vi "PathDrawerMain.vi"() -> ()   [LabVIEW 2017]
uses:
  Shared/PathFileData.ctl
  Shared/RobotNeededPathData.ctl
panel:
  in  "Tab Control":enum32{"Path", "Load/Save"}(tab)
  in  "SlowSpeed":dbl=15.0 format="%#_13g"
  in  "SlowDistanceAtEnd":dbl=12.0 format="%#_13g"
  in  "Speed/Curve":dbl=1.8 format="%#_13g"
  in  "DriveBackwards?":bool
  in  "Lookahead":dbl=15.0
  out "Points (in)":cluster{dbl, dbl}[](array[cluster])=[{10.226685796269727, 128.2984218077475}, {15.522939790252737, 129.12001667538078}, {20.706046011417115, 130.03734410344734}, {25.64419820355277, 131.16153224586634}, {30.166489666811938, 132.63728713251658}, {34.03433393234178, 134.66614678695453}, {37.84312996845399, 137.57541844379503}, {41.613199324830866, 141.06936663595954}, {45.358528302145274, 144.94685599230576}, {49.089111176273455, 149.06887095200779}, {52.81248148388562, 153.3359781588411}, {56.53509433279494, 157.67228944092315}, {60.26328881425947, 162.01308055786865}, {64.00426865578318, 166.29432163323958}, {67.7673029921362, 170.44235444566638}, {71.56524618905358, 174.36196698028664}, {75.41661103612846, 177.92096482194324}, {79.3485578107416, 180.92876767612321}, {83.40129053463254, 183.10555843063264}, {88.0121428846403, 184.52243744962843}, {92.95651186406619, 185.43308931394066}, {98.06376666039486, 186.00922465888777}, {103.18969721381382, 186.36840832003176}, {108.19306201885799, 186.59306844321625}, {112.91282926380357, 186.74384781305636}, {117.14203730272597, 186.86944045911048}]
  in  "Points":cluster{dbl, dbl}[](array[cluster])=[{35.0, 207.0}, {61.0, 206.0}, {110.0, 143.0}, {150.0, 144.0}]
  in  "Roundedness":dbl(slide)=0.8606565656565657 scale=0.6..0.997
  in  "Length":dbl=29.0
  in  "Width":dbl=32.0
  in  "CenterRotOffset":dbl=10.5
  in  "PointSpacing":dbl=6.0 min=1.0 format="%#_13g"
  in  "StartingPosition":enum16{"1", "2", "3", "4", "No Preset"}(ring)=enum."3"
  in  "Flip Path":bool
  in  "MaxVel":dbl=130.0 format="%#_13g"
  in  "MaxAccel":dbl=50.0 format="%#_13g"
  in  "ExportAllToRobot":bool
  in  "LocalTempPaths":i32(listbox)
  out "standard output":string
  in  "SaveToLocal":bool
  in  "LoadFromLocal":bool
  in  "ExportToRobot":bool
  in  "LoadAllFromRobot":bool
  in  "LocalPaths":i32(listbox)=3
  out "standard error":string="NI Linux Real-Time (run mode)\n\nLog in with your NI-Auth credentials.\n\n"
  in  "LocalFileNames":string[](array[string])=["1A.txt", "1B.txt", "1C.txt", "3A.txt", "4B.txt"]
  in  "Stop":bool
  out "Path Drawer":T1(plugin-control)
  # "Includes bumpers"
  # "Relative to outside face of\nback bumber of robot"
  # "INSTRUCTIONS"
  # "The red line is the path that the robot recieves. Everything else is to help create that path\n\nUse the multi-line tool to draw a path. Double click to stop drawing.\nHover over a node and press backspace to remove it.\nPress I to insert a new node (at the end of the path only, for now)\n\nUse the contols to input robot width, height, and center of rotation offset,\nHow far apart the points in the \"real world units\" path are,\nWhether the robot travels on the left or right of your green lines, and\nthe roundedness of the path. (Note: point spacing affects roundedness)\n\nYou can manually edit the green node's location in the path with the Points array,\nor drag the nodes on the image\n\nPress Export To File and enter the file name (no extension) to save the path to a file in the\nThisVIsDirectory\\Paths\\ folder\n\nIf you acidentally clear your path press Z quickly to get it back"
  # "Responses of CMDs run"
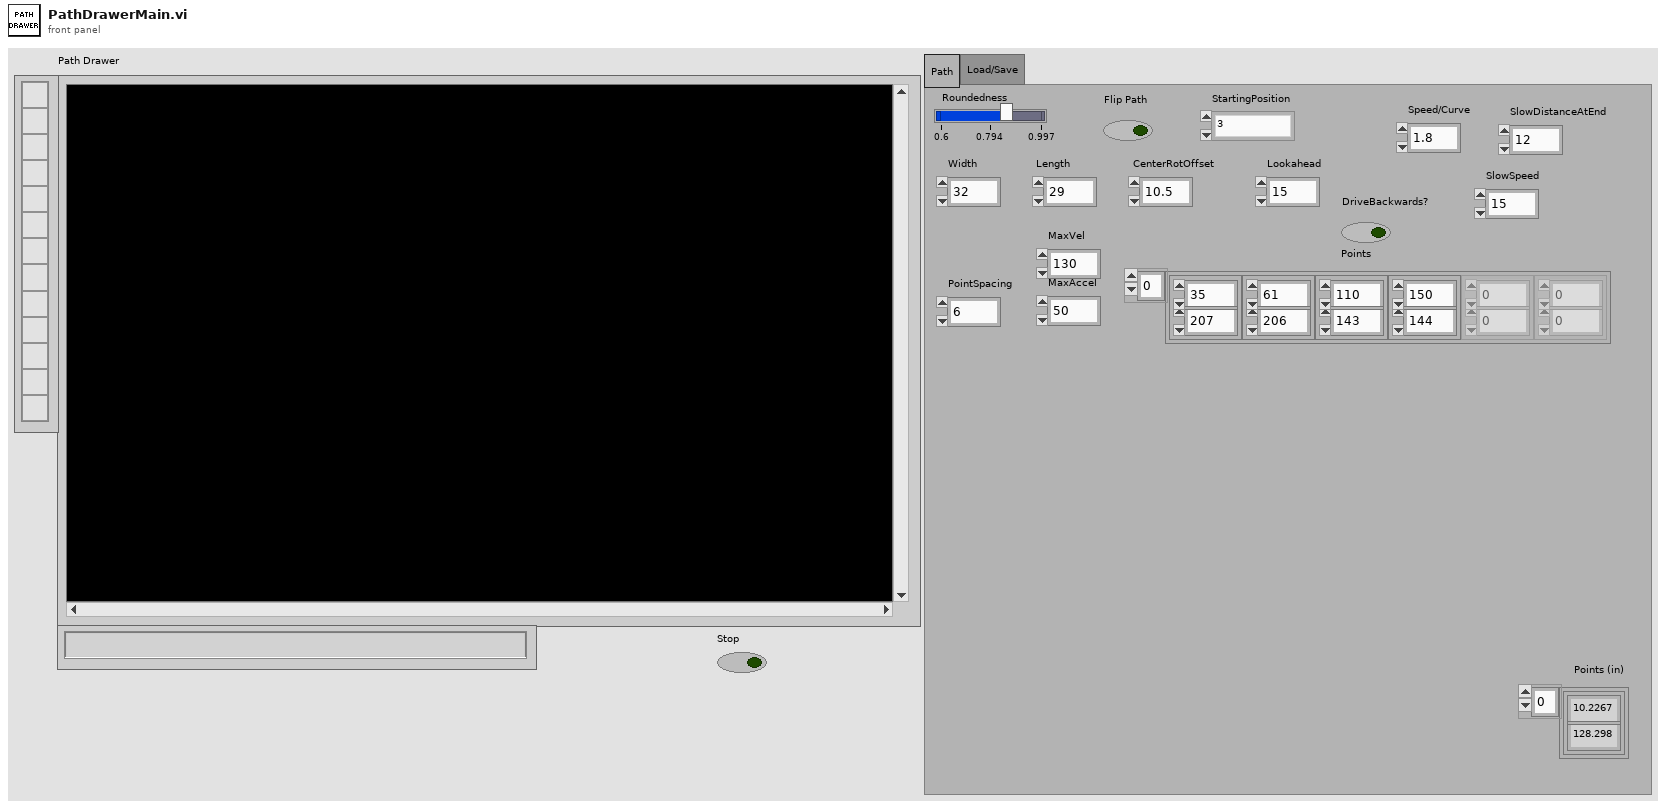
[diagram p1: front panel]
types:
  T1 = typedef "IMAQ Image.ctl" = refnum<image>
  T2 = typedef "Image Type" = u32
  T3 = enum16{"open", "replace", "create", "open or create", "replace or create", "replace or create with confirmation"}
  T4 = cluster{"Global Rectangle":i32[], "Contours":cluster{"Contour Type":u32, "ROI Type":u32, "Points":i32[]}[]}
  T5 = cluster{"Contour Type":u32, "ROI Type":u32, "Points":i32[]}[]
  T6 = cluster{"Contour Type":u32, "ROI Type":u32, "Points":i32[]}
  T7 = typedef "PathFileData.ctl" = cluster{"RobotNeeded":T8, "Meta":cluster{"Path (px)":cluster{i32, i32}[], "RobotWidth":dbl, "RobotLength":dbl, "CenterOfRotYOffset":dbl, "Roundedness":dbl, "StartingPositionPreset":u32, "PathName":string}}
  T8 = typedef "RobotNeededPathData.ctl" = cluster{"Path":cluster{dbl, dbl}[], "MaxVel":dbl, "MaxAccel":dbl, "Backwards?":bool, "PointSpacing":dbl, "LookaheadDist":dbl, "Speed/Curve":dbl, "SlowDistanceAtEnd":dbl, "SlowSpeed":dbl}
  T9 = cluster{"Path (px)":cluster{i32, i32}[], "RobotWidth":dbl, "RobotLength":dbl, "CenterOfRotYOffset":dbl, "Roundedness":dbl, "StartingPositionPreset":u32, "PathName":string}
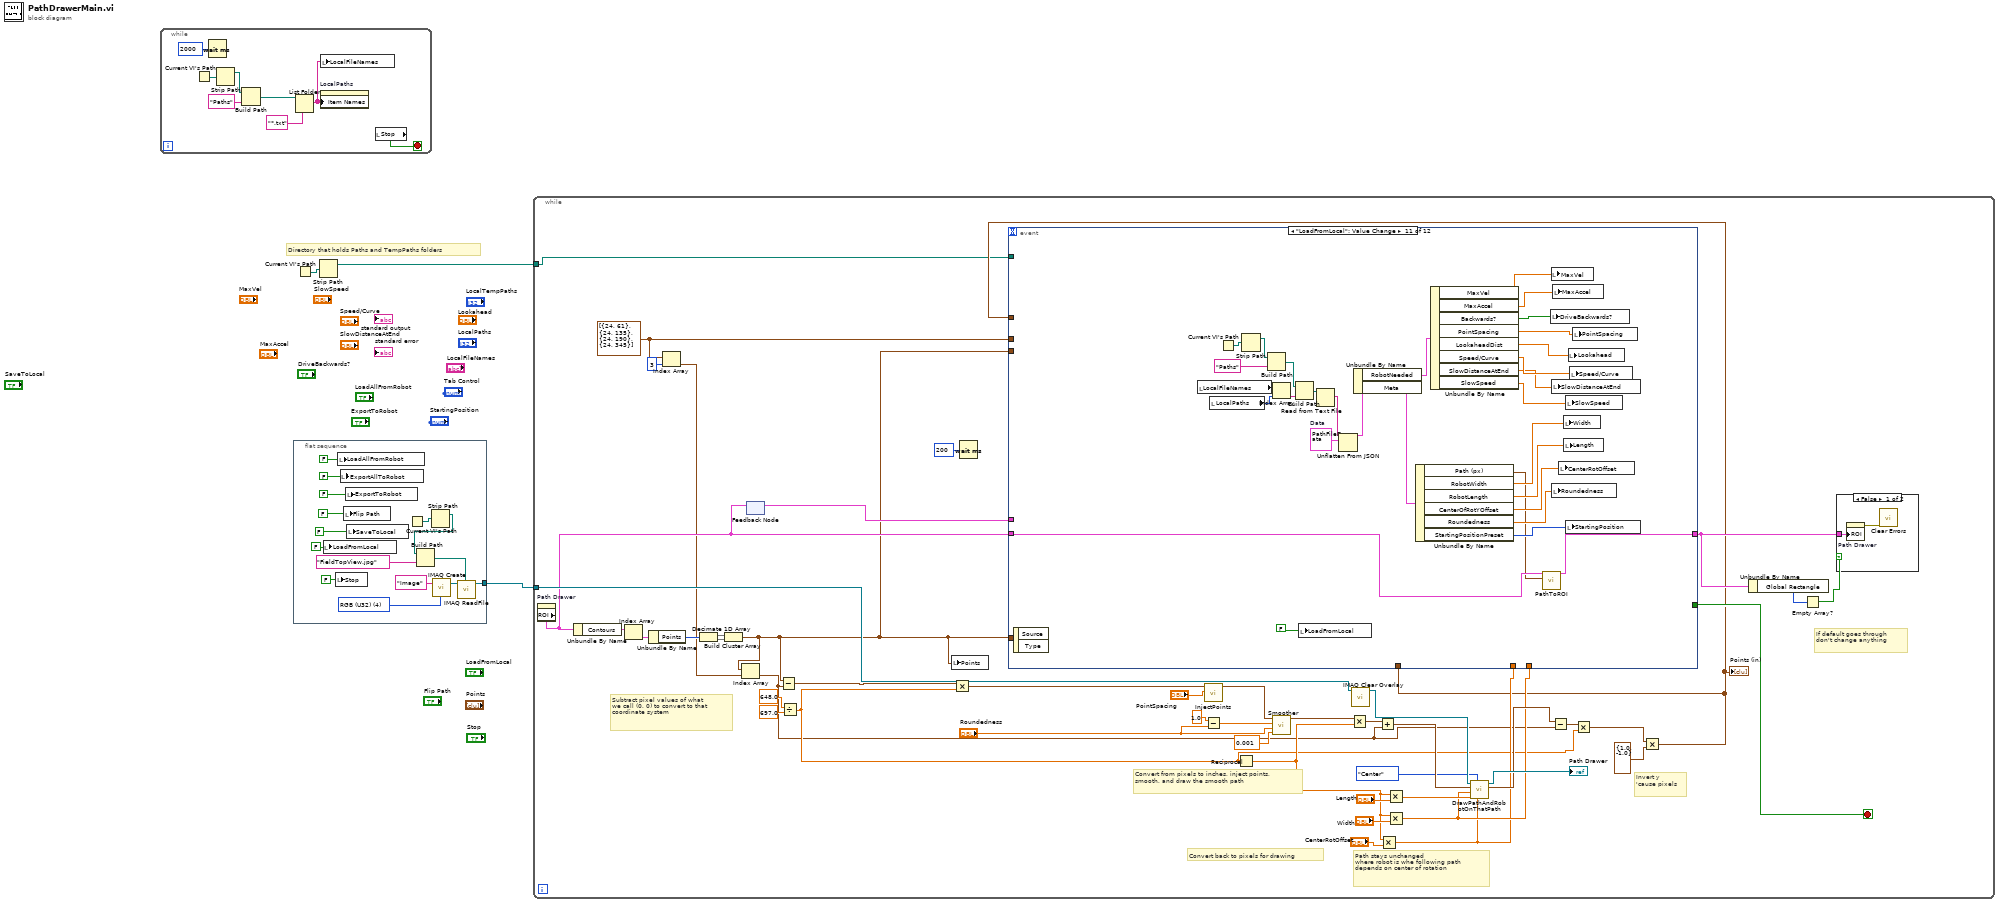
[diagram p0: block diagram]
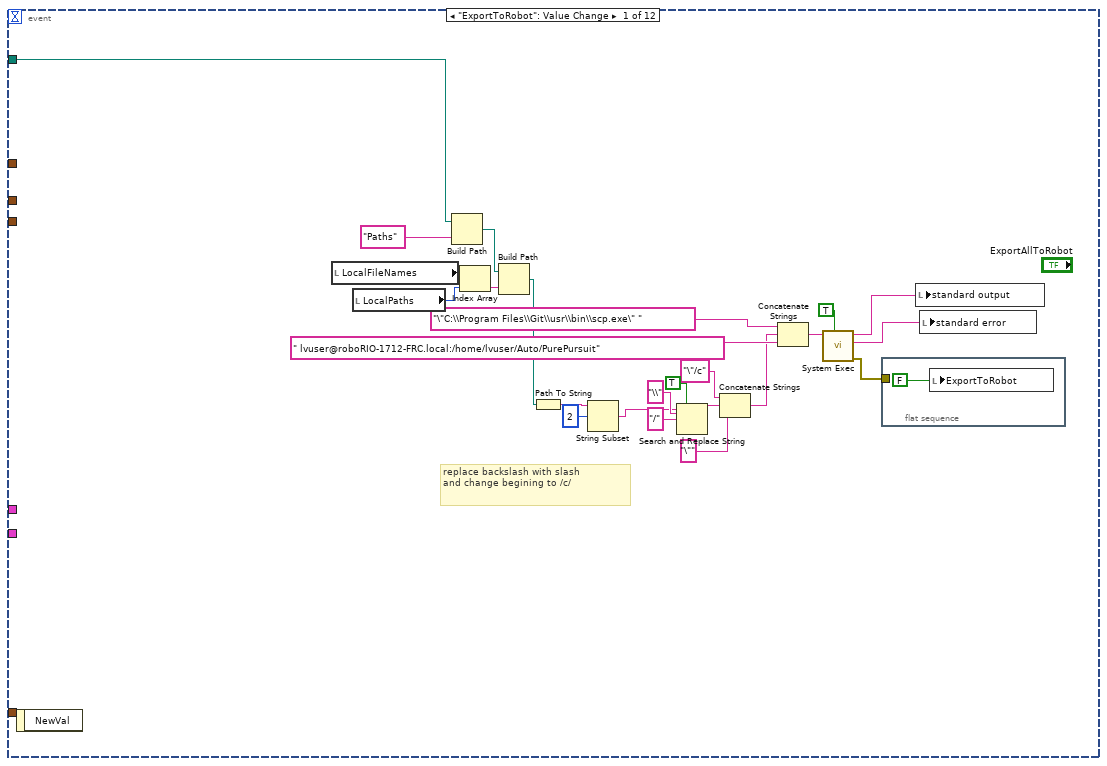
[diagram p3: hidden frame]
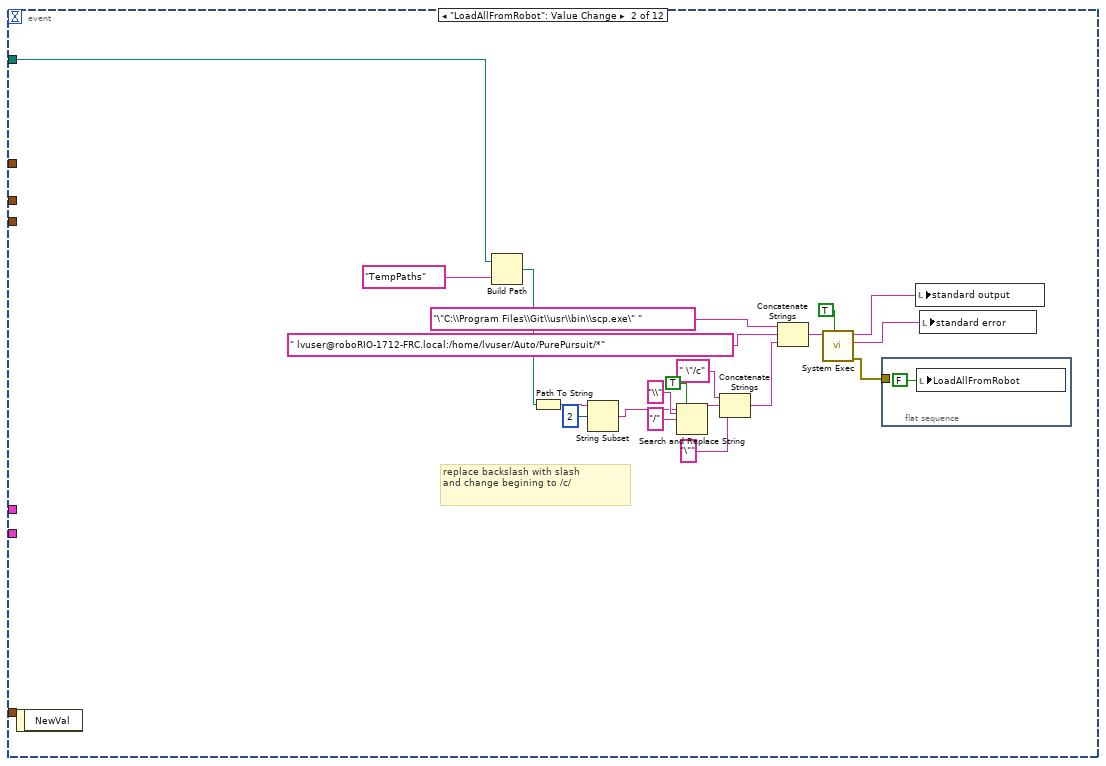
[diagram p4: hidden frame]
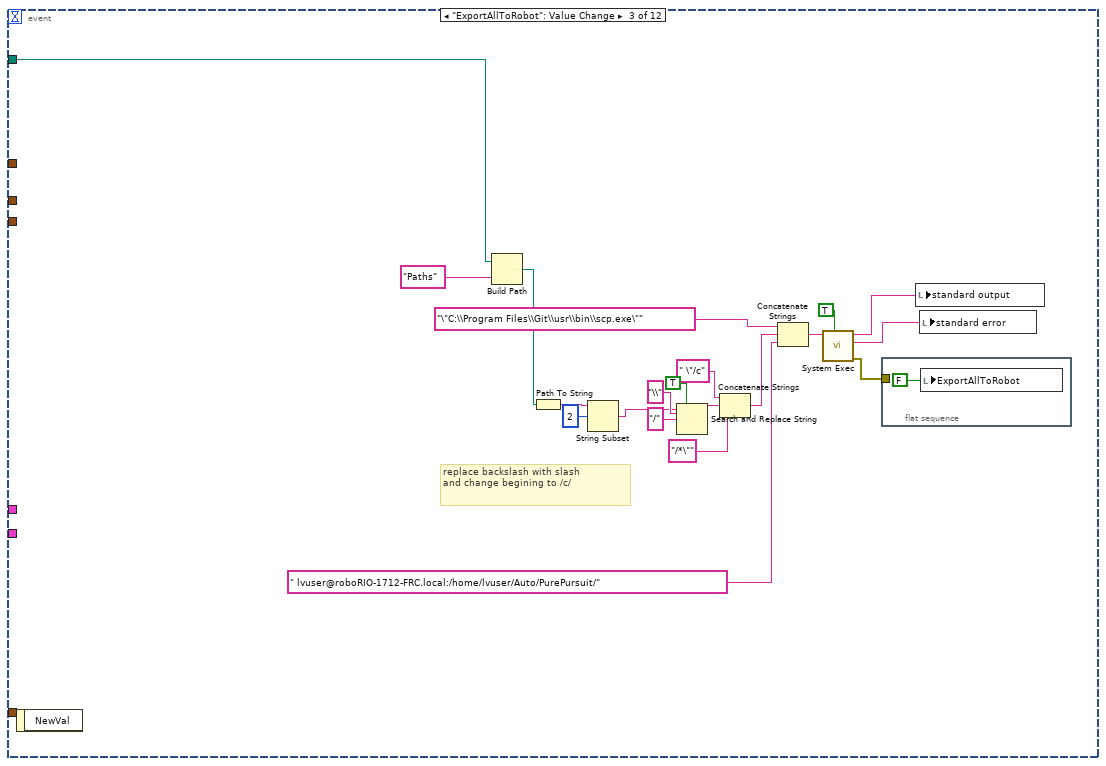
[diagram p5: hidden frame]
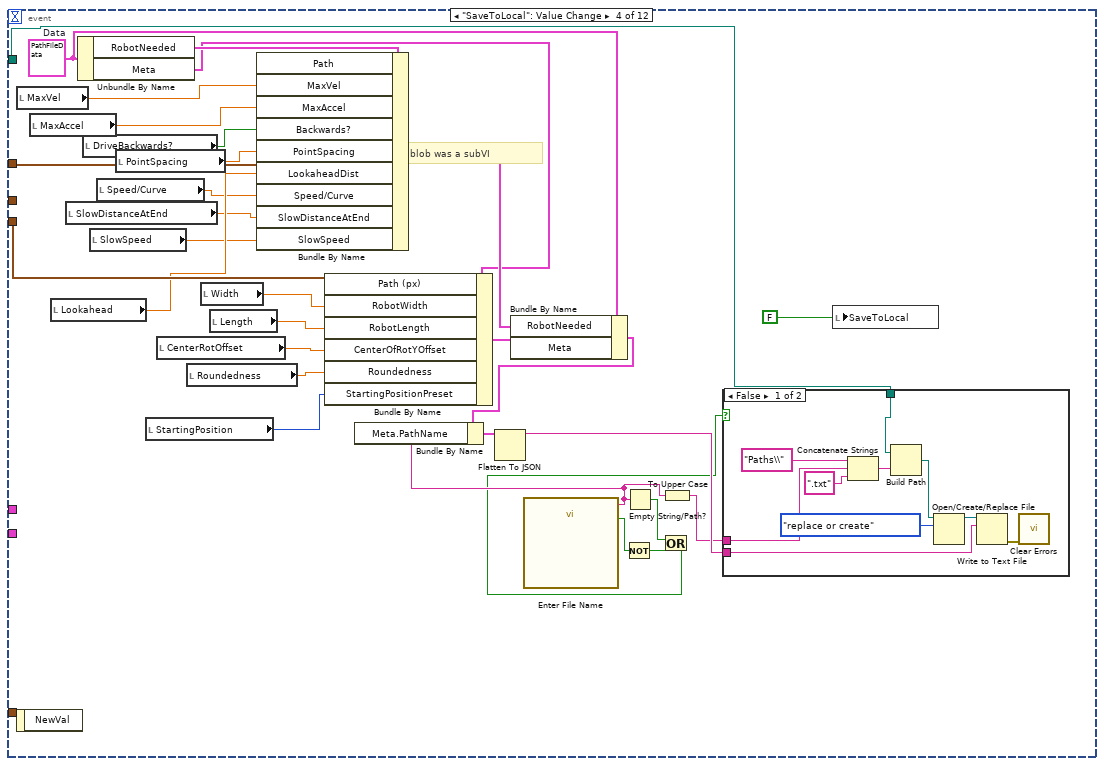
[diagram p6: hidden frame]
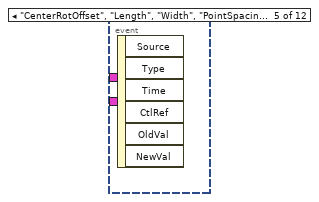
[diagram p8: hidden frame]
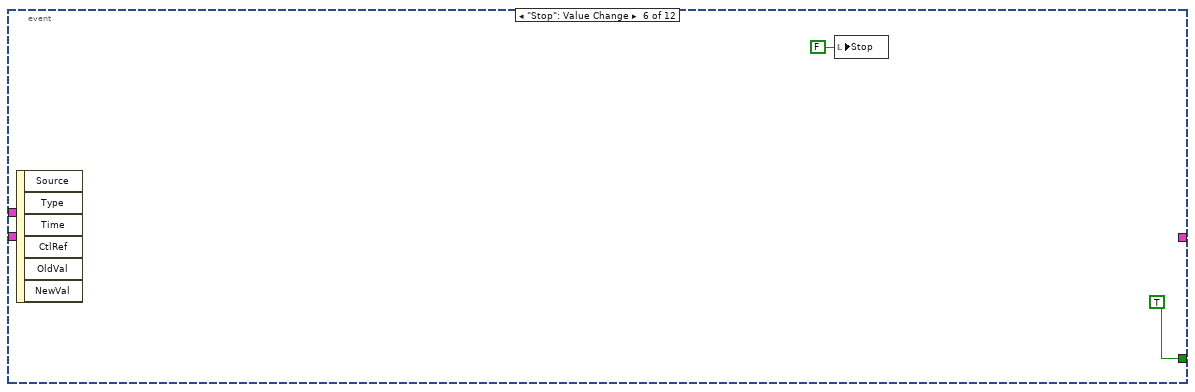
[diagram p9: hidden frame]
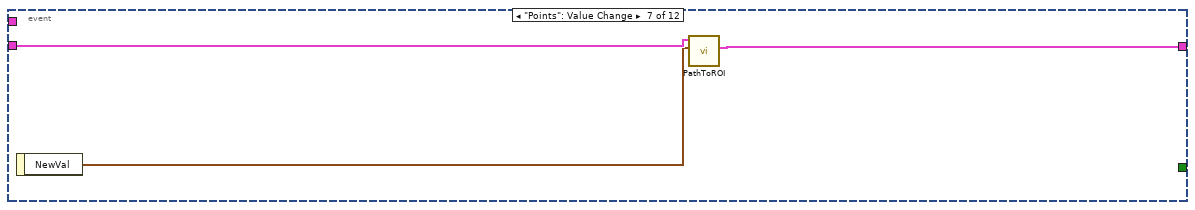
[diagram p10: hidden frame]
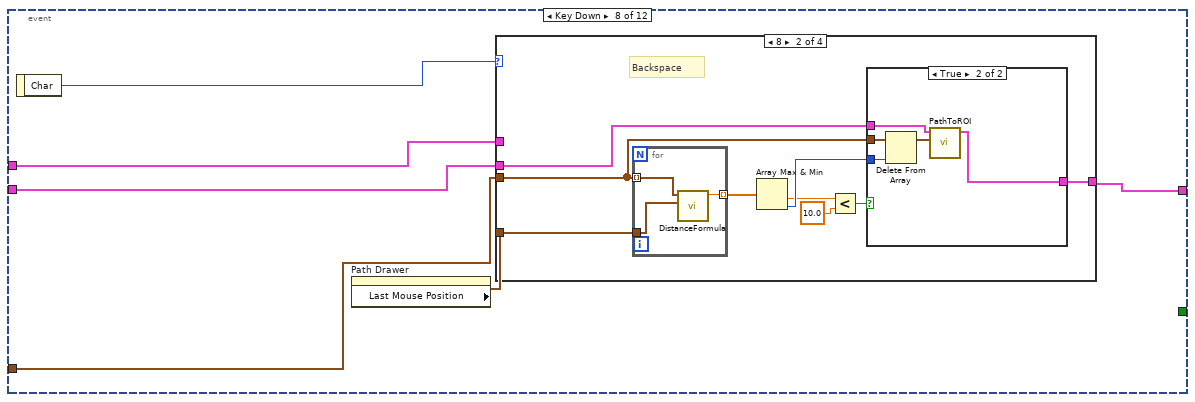
[diagram p11: hidden frame]
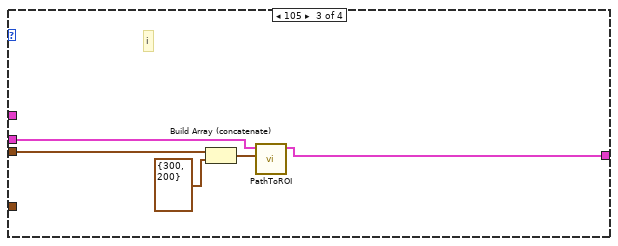
[diagram p14: hidden frame]
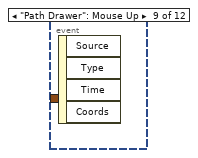
[diagram p16: hidden frame]
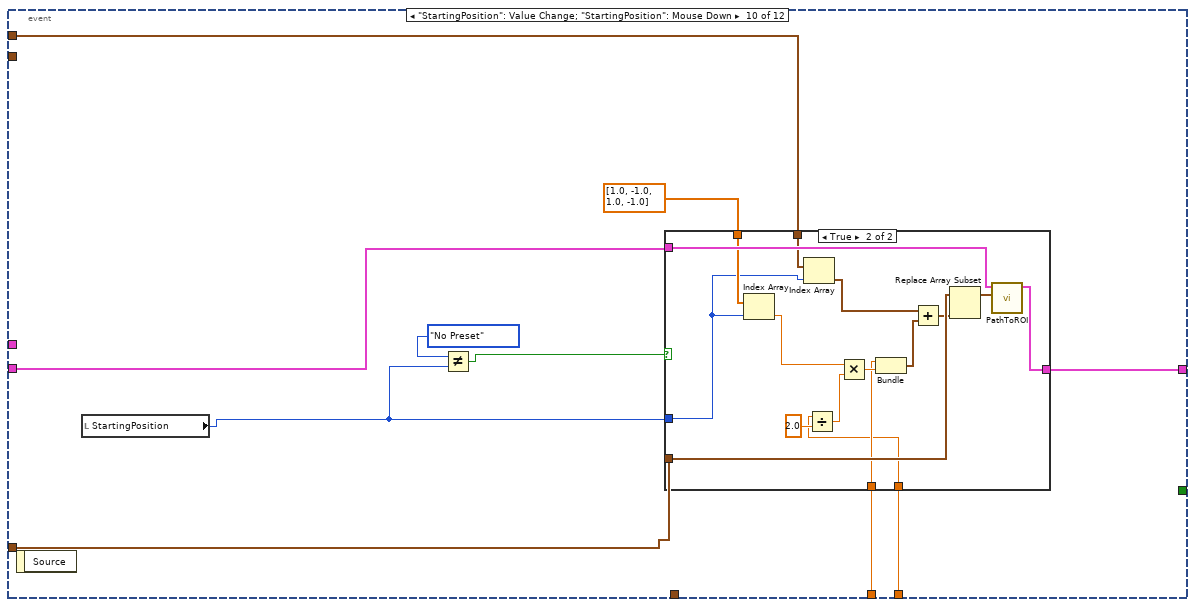
[diagram p17: hidden frame]
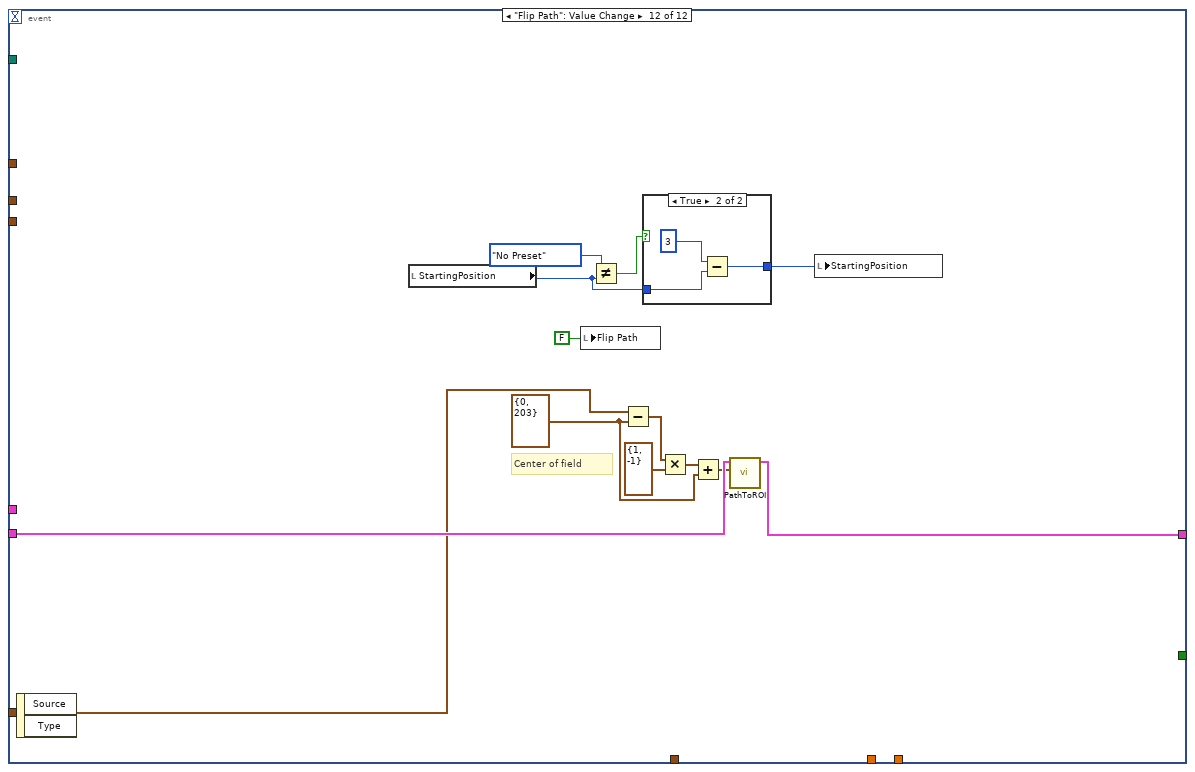
[diagram p19: hidden frame]
diagram:
  # "Directory that holds Paths and TempPaths folders"
  n1 = while {
    stop <- w10 stop-if-true
    n2 = Current VI's Path() -> (path=w5:path)
    n3 = Wait (ms)(milliseconds to wait=u32 2000) -> ()  [unwired: 1 out]
    n4 = Strip Path(path=w5) -> (stripped path=w4:path)  [unwired: 1 out]
    n5 = Build Path(base path=w4, name or relative path="Paths") -> (appended path=w7:path)
    n6 = List Folder(path=w7, pattern="*.txt") -> (filenames=w9:string[])  [unwired: 2 in, 3 out]
    n7 = local write "LocalFileNames"(w9) -> ()
    n8 = property on="LocalPaths" class="LstBox (strict)"("Item Names"=w9) -> ()  [unwired: 2 in, 2 out]
    n9 = local read "Stop"() -> (w10:bool)
  }
  n10 = flat-sequence {
    tunnel: [w21] -> w3
    frame #0 {
      w23 = T2 4 items=["Grayscale (U8)", "Grayscale (I16)", "Grayscale (SGL)", "Complex (CSG)", "RGB (U32)", "HSL (U32)", "RGB (U64)", "Grayscale (U16)"] ("Image Type")
      n11 = local write "LoadFromLocal"(FALSE ("Export To File")) -> ()
      n12 = local write "Stop"(FALSE ("Stop")) -> ()
      n13 = local write "LoadAllFromRobot"(FALSE ("Export To File")) -> ()
      n14 = local write "ExportAllToRobot"(FALSE ("Export To File")) -> ()
      n15 = local write "Flip Path"(FALSE ("Export To File")) -> ()
      n16 = local write "ExportToRobot"(FALSE ("Export To File")) -> ()
      n17 = local write "SaveToLocal"(FALSE ("Export To File")) -> ()
      n18 = Current VI's Path() -> (path=w15:path)
      n19 = Strip Path(path=w15) -> (stripped path=w14:path)  [unwired: 1 out]
      n20 = Build Path(base path=w14, name or relative path="FieldTopView.jpg") -> (appended path=w25:path)
      n21 = call "IMAQ Create"("Image Name"="Image", "Image Type"=w23) -> ("New Image"=w22:T1)  [unwired: 3 in, 1 out]
      n22 = call "IMAQ ReadFile"("File Path"=w25, "Image"=w22) -> ("Image Out"=w21:T1)  [unwired: 5 in, 4 out]
    }
  }
  n23 = Current VI's Path() -> (path=w2:path)
  n24 = Strip Path(path=w2) -> (stripped path=w1:path)  [unwired: 1 out]
  n25 = while {
    tunnel: w3 -> [w67]
    tunnel: w1 -> [w30]
    stop <- w40 stop-if-true
    w29 = cluster{u32, u32}[] [{24, 61}, {24, 135}, {24, 190}, {24, 345}]
    # "Invert y\n'cause pixels"
    # "Path stays unchanged\nwhere robot is whe following path\ndepends on center of rotation"
    # "Convert back to pixels for drawing"
    # "If default goes through\ndon't change anything"
    # "Convert from pixels to inches, inject points,\nsmooth, and draw the smooth path"
    # "Subtract pixel values of what\nwe call (0, 0) to convert to that\ncoordinate system"
    n26 = property on="Path Drawer" class="ImageControl"() -> ("ROI"=w34:T4)  [unwired: 2 in, 2 out]
    n27 = Unbundle By Name(w34) -> ("Contours"=w73:T5)
    n28 = Index Array(array=w73) -> (element=w68:T6)  [unwired: 1 in]
    n29 = Unbundle By Name(w68) -> ("Points"=w62:i32[])
    n30 = Index Array(array=w29, index=3) -> (element=w27:cluster{u32, u32})
    n31 = Decimate 1D Array(w62) -> (w72:i32[], w71:i32[])
    n32 = Build Cluster Array(w72, w71) -> (w32:cluster{i32, i32}[])
    n33 = Index Array(array=w32) -> ()  [unwired: 1 in, 1 out]
    n34 = feedback-in #1(w34) -> ()
    n35 = feedback #1() -> (w49:T4)  [unwired: 1 in]
    n36 = Subtract(x=w32, y=w27) -> (x-y=w63:cluster{u32, u32}[])
    n37 = Divide(x=648.0, y=697.0) -> (x/y=w35:dbl)
    n38 = local write "Points"(w32) -> ()
    n39 = Multiply(x=w63, y=w35) -> (x*y=w50:cluster{dbl, dbl}[])
    n40 = Wait (ms)(milliseconds to wait=u32 200) -> ()  [unwired: 1 out]
    n41 = call "InjectPoints.vi"("Distance"="PointSpacing", "Path"=w50) -> ("Path out"=w65:cluster{dbl, dbl}[])  [unwired: 9 in]
    n42 = Subtract(x=1.0, y="Roundedness") -> (x-y=w60:dbl)
    n43 = Reciprocal(x=w35) -> (1/x=w47:dbl)
    n44 = call "Smoother.vi"("tolerance"=0.001, "B"="Roundedness", "A"=w60, "Path"=w65) -> ("SmoothPath"=w55:cluster{dbl, dbl}[])  [unwired: 7 in]
    n45 = Multiply(x=w55, y=w47) -> (x*y=w64:cluster{dbl, dbl}[])
    n46 = call "IMAQ Clear Overlay"("Image"=w67) -> ("Image Out"=w44:T1)  [unwired: 9 in, 1 out]
    n47 = Add(x=w64, y=w27) -> (x+y=w43:cluster{dbl, dbl}[])
    n48 = Multiply(x=w47, y="CenterRotOffset") -> (x*y=w38:dbl)
    n49 = Multiply(x=w47, y="Length") -> (x*y=w42:dbl)
    n50 = Multiply(x=w47, y="Width") -> (x*y=w39:dbl)
    n51 = call "DrawPathAndRobotOnThatPath.vi"("CenterOfRotYOffset (px)"=w38, "PathMode"=enum16{"Left", "Right", "Center"}."Center", "RobotLength (px)"=w42, "RobotWidth (px)"=w39, "Path (px)"=w43, "Image In"=w44) -> ("NewPath (px)"=w45:cluster{dbl, dbl}[], "Image Out"=→"Path Drawer":T1)  [unwired: 4 in]
    n52 = Subtract(x=w45, y=w27) -> (x-y=w51:cluster{dbl, dbl}[])
    n53 = Multiply(x=w51, y=w35) -> (x*y=w37:cluster{dbl, dbl}[])
    n54 = Multiply(x=w37, y=cluster{dbl, dbl} {1.0, -1.0}) -> (x*y=w31:cluster{dbl, dbl}[])
    "Points (in)" <- w31
    n55 = event shown="[10] \"LoadFromLocal\": Value Change" {
      selector: _ -> [_ _ _ _ _ _ _ _ _ _ _ _]
      dyn-events: _ -> [_ _ _ _ _ _ _ _ _ _ _ _]
      timeout: _ -> [_ _ _ _ _ _ _ _ _ _ _ _]
      tunnel: w34 -> [_ _ _ _ _ _ w188 w194 _ w228 w260 w287]
      tunnel: [_ _ _ _ _ _ w187 w191 _ w229 w274 w286] -> w33
      tunnel: w31 -> [_ _ _ _ _ _ _ _ _ _ _ _]
      tunnel: w49 -> [_ _ _ _ _ _ _ w190 _ _ _ _]
      tunnel: w32 -> [_ _ _ _ _ _ _ w189 _ w223 _ w281]
      tunnel: w38 -> [_ _ _ _ _ _ _ _ _ w225 _ _]
      tunnel: w39 -> [_ _ _ _ _ _ _ _ _ w224 _ _]
      tunnel: [_ _ _ _ _ TRUE ("Stop") _ _ _ _ _ _] -> w40
      tunnel: w32 -> [_ _ _ w157 _ _ _ _ _ _ _ _]
      tunnel: w31 -> [_ _ _ w156 _ _ _ _ _ _ _ _]
      tunnel: w30 -> [w76 w101 w122 w149 _ _ _ _ _ _ _ _]
      tunnel: w29 -> [_ _ _ _ _ _ _ _ _ w220 _ _]
      event "ExportToRobot": Value Change {
        # "replace backslash with slash\nand change begining to /c/"
        n56 = event-data() -> ()  [unwired: 1 in, 1 out]
        n57 = local read "LocalFileNames"() -> (w83:string[])
        n58 = local read "LocalPaths"() -> (w84:i32)
        n59 = Build Path(base path=w76, name or relative path="Paths") -> (appended path=w86:path)
        n60 = Index Array(array=w83, index=w84) -> (element=w85:string)
        n61 = Build Path(base path=w86, name or relative path=w85) -> (appended path=w81:path)
        n62 = Path To String(path=w81) -> (string=w92:string)
        n63 = String Subset(string=w92, offset (0)=2) -> (substring=w90:string)  [unwired: 1 in]
        n64 = Search and Replace String(replace all?=TRUE ("replace all? (F)"), input string=w90, search string="\\", replace string="/" ("replace string (\"\")")) -> (result string=w89:string)  [unwired: 4 in, 3 out]
        n65 = Concatenate Strings("\"/c" ("string"), w89, "\"" ("string")) -> (w87:string)
        n66 = Concatenate Strings("\"C:\\Program Files\\Git\\usr\\bin\\scp.exe\" " ("command line"), w87, " lvuser@roboRIO-1712-FRC.local:/home/lvuser/Auto/PurePursuit" ("string")) -> (w96:string)
        n67 = call <vilib>:"System Exec.vi"("wait until completion? (T)"=TRUE, "command line"=w96) -> ("error out"=w79:errorcluster, "standard error"=w77:string, "standard output"=w78:string)  [unwired: 6 in, 1 out]
        n68 = flat-sequence {
          tunnel: w79 -> [_]
          frame #0 {
            n69 = local write "ExportToRobot"(FALSE ("Export To File")) -> ()
          }
        }
        n70 = local write "standard output"(w78) -> ()
        n71 = local write "standard error"(w77) -> ()
      }
      event "LoadAllFromRobot": Value Change {
        # "replace backslash with slash\nand change begining to /c/"
        n72 = event-data() -> ()  [unwired: 1 in, 1 out]
        n73 = Build Path(base path=w101, name or relative path="TempPaths") -> (appended path=w104:path)
        n74 = Path To String(path=w104) -> (string=w114:string)
        n75 = String Subset(string=w114, offset (0)=2) -> (substring=w112:string)  [unwired: 1 in]
        n76 = Search and Replace String(replace all?=TRUE ("replace all? (F)"), input string=w112, search string="\\", replace string="/" ("replace string (\"\")")) -> (result string=w111:string)  [unwired: 4 in, 3 out]
        n77 = Concatenate Strings(" \"/c" ("string"), w111, "\"" ("string")) -> (w102:string)
        n78 = Concatenate Strings("\"C:\\Program Files\\Git\\usr\\bin\\scp.exe\" " ("command line"), " lvuser@roboRIO-1712-FRC.local:/home/lvuser/Auto/PurePursuit/*" ("string"), w102) -> (w118:string)
        n79 = call <vilib>:"System Exec.vi"("wait until completion? (T)"=TRUE, "command line"=w118) -> ("error out"=w107:errorcluster, "standard error"=w105:string, "standard output"=w106:string)  [unwired: 6 in, 1 out]
        n80 = flat-sequence {
          tunnel: w107 -> [_]
          frame #0 {
            n81 = local write "LoadAllFromRobot"(FALSE ("Export To File")) -> ()
          }
        }
        n82 = local write "standard output"(w106) -> ()
        n83 = local write "standard error"(w105) -> ()
      }
      event "ExportAllToRobot": Value Change {
        # "replace backslash with slash\nand change begining to /c/"
        n84 = event-data() -> ()  [unwired: 1 in, 1 out]
        n85 = Build Path(base path=w122, name or relative path="Paths") -> (appended path=w125:path)
        n86 = Path To String(path=w125) -> (string=w135:string)
        n87 = String Subset(string=w135, offset (0)=2) -> (substring=w133:string)  [unwired: 1 in]
        n88 = Search and Replace String(replace all?=TRUE ("replace all? (F)"), input string=w133, search string="\\", replace string="/" ("replace string (\"\")")) -> (result string=w132:string)  [unwired: 4 in, 3 out]
        n89 = Concatenate Strings(" \"/c" ("string"), w132, "/*\"" ("string")) -> (w124:string)
        n90 = Concatenate Strings("\"C:\\Program Files\\Git\\usr\\bin\\scp.exe\"" ("command line"), w124, " lvuser@roboRIO-1712-FRC.local:/home/lvuser/Auto/PurePursuit/" ("string")) -> (w139:string)
        n91 = call <vilib>:"System Exec.vi"("wait until completion? (T)"=TRUE, "command line"=w139) -> ("error out"=w128:errorcluster, "standard error"=w126:string, "standard output"=w127:string)  [unwired: 6 in, 1 out]
        n92 = flat-sequence {
          tunnel: w128 -> [_]
          frame #0 {
            n93 = local write "ExportAllToRobot"(FALSE ("Export To File")) -> ()
          }
        }
        n94 = local write "standard output"(w127) -> ()
        n95 = local write "standard error"(w126) -> ()
      }
      event "SaveToLocal": Value Change {
        w155 = T7 {"RobotNeeded"={"Path"=[], "MaxVel"=0.0, "MaxAccel"=0.0, "Backwards?"=FALSE, "PointSpacing"=0.0, "LookaheadDist"=0.0, "Speed/Curve"=1.8, "SlowDistanceAtEnd"=12.0, "SlowSpeed"=15.0}, "Meta"={"Path (px)"=[], "RobotWidth"=0.0, "RobotLength"=0.0, "CenterOfRotYOffset"=0.0, "Roundedness"=0.0, "StartingPositionPreset"=2, "PathName"=""}}  # Data
        # "I wish this blob was a subVI"
        n96 = local read "MaxVel"() -> (w148:dbl)
        n97 = event-data() -> ()  [unwired: 1 in, 1 out]
        n98 = local read "MaxAccel"() -> (w147:dbl)
        n99 = local read "Lookahead"() -> (w151:dbl)
        n100 = local read "SlowDistanceAtEnd"() -> (w144:dbl)
        n101 = Unbundle By Name(w155) -> ("RobotNeeded"=w164:T8, "Meta"=w163:T9)
        n102 = local read "DriveBackwards?"() -> (w150:bool)
        n103 = local read "SlowSpeed"() -> (w143:dbl)
        n104 = local read "Speed/Curve"() -> (w145:dbl)
        n105 = local read "PointSpacing"() -> (w167:dbl)
        n106 = local read "StartingPosition"() -> (w166:enum16{"1", "2", "3", "4", "No Preset"})
        n107 = local read "CenterRotOffset"() -> (w159:dbl)
        n108 = local read "Roundedness"() -> (w158:dbl)
        n109 = local read "Width"() -> (w161:dbl)
        n110 = local read "Length"() -> (w160:dbl)
        n111 = Bundle By Name(cluster=w164, "Path"=w156, "MaxVel"=w148, "MaxAccel"=w147, "Backwards?"=w150, "PointSpacing"=w167, "LookaheadDist"=w151, "Speed/Curve"=w145, "SlowDistanceAtEnd"=w144, "SlowSpeed"=w143) -> (w165:T8)
        n112 = Bundle By Name(cluster=w163, "Path (px)"=w157, "RobotWidth"=w161, "RobotLength"=w160, "CenterOfRotYOffset"=w159, "Roundedness"=w158, "StartingPositionPreset"=w166) -> (w162:T9)
        n113 = Bundle By Name(cluster=w155, "RobotNeeded"=w165, "Meta"=w162) -> (w154:T7)
        n114 = call "Enter File Name"() -> ("File Name"=w153:string, "Enter"=w169:bool)  [unwired: 17 in, 1 out]
        n115 = Bundle By Name(cluster=w154, "Meta.PathName"=w153) -> (w171:T7)
        n116 = Flatten To JSON(anything=w171) -> (JSON string=w172:string)  [unwired: 2 in, 1 out]
        n117 = Not(x=w169) -> (.not. x?=w168:bool)
        n118 = Empty String/Path?(string/path=w153) -> (empty?=w170:bool)
        n119 = Or(x=w170, y=w168) -> (x .or. y?=w146:bool)
        n120 = To Upper Case(1:w153) -> (0:w152:string)
        n121 = case shown="False" w146 {
          tunnel: w152 -> [w179 _]
          tunnel: w172 -> [w178 _]
          tunnel: w149 -> [w174 _]
          frame False {
            n122 = Concatenate Strings("Paths\\" ("name or relative path"), w179, ".txt" ("string")) -> (w183:string)
            n123 = Build Path(base path=w174, name or relative path=w183) -> (appended path=w177:path)
            n124 = Open/Create/Replace File(file path (use dialog)=w177, operation (0:open)=T3."replace or create") -> (refnum out=w176:refnum<file>)  [unwired: 4 in, 2 out]
            n125 = Write to Text File(file (use dialog)=w176, text=w178) -> (error out=w181:errorcluster)  [unwired: 2 in, 2 out]
            n126 = call <vilib>:"Clear Errors.vi"("error in (no error)"=w181) -> ()  [unwired: 5 in, 2 out]
          }
          frame True {
          }
        }
        n127 = local write "SaveToLocal"(FALSE ("Export To File")) -> ()
      }
      event "CenterRotOffset", "Length", "Width", "PointSpacing", "Roundedness": Value Change {
        n128 = event-data() -> ()  [unwired: 1 in, 6 out]
      }
      event "Stop": Value Change {
        n129 = event-data() -> ()  [unwired: 1 in, 6 out]
        n130 = local write "Stop"(FALSE ("Stop")) -> ()
      }
      event "Points": Value Change {
        n131 = event-data() -> ("NewVal"=w186:cluster{dbl, dbl}[])  [unwired: 1 in]
        n132 = call "PathToROI.vi"("Path In"=w186, "ROI In"=w188) -> ("ROI Out"=w187:T4)  [unwired: 9 in]
      }
      event Key Down {
        n133 = event-data() -> ("Char"=w193:i16)  [unwired: 1 in]
        n134 = property on="Path Drawer" class="ImageControl"() -> ("Last Mouse Position"=w192:cluster{"X":i32, "Y":i32})  [unwired: 2 in, 2 out]
        n135 = case shown="8" w193 {
          tunnel: w194 -> [w195 w204 w216 _]
          tunnel: w189 -> [_ w203 w218 _]
          tunnel: w192 -> [_ w197 _ _]
          tunnel: [w195 w196 w214 w219] -> w191
          tunnel: w190 -> [_ _ _ w219]
          frame 0, Default {
          }
          frame 8 {
            # "Backspace"
            n136 = for {
              tunnel: w203 -> [w213] mode=indexing
              tunnel: [w212] -> w202 mode=indexing
              tunnel: w197 -> [w211]
              n137 = call "DistanceFormula.vi"("Point 2"=w211, "Point 1"=w213) -> ("Distance"=w212:dbl)  [unwired: 9 in]
            }
            n138 = Array Max & Min(array=w202) -> (min value=w200:dbl, min index (indices)=w201:i32)  [unwired: 2 out]
            n139 = Less?(x=w200, y=10.0) -> (x < y?=w198:bool)
            n140 = case shown="True" w198 {
              tunnel: w201 -> [_ w210]
              tunnel: w203 -> [_ w209]
              tunnel: w204 -> [w205 w207]
              tunnel: [w205 w206] -> w196
              frame False {
              }
              frame True {
                n141 = Delete From Array(array=w209, index=w210) -> (array with subset deleted=w208:cluster{i32, i32}[])  [unwired: 1 in, 1 out]
                n142 = call "PathToROI.vi"("Path In"=w208, "ROI In"=w207) -> ("ROI Out"=w206:T4)  [unwired: 9 in]
              }
            }
          }
          frame 105 {
            # "i"
            n143 = Build Array (concatenate)(w218, cluster{i32, i32} {300, 200}) -> (w217:cluster{i32, i32}[])
            n144 = call "PathToROI.vi"("Path In"=w217, "ROI In"=w216) -> ("ROI Out"=w214:T4)  [unwired: 9 in]
          }
          frame 122 {
            # "Restore last ROI"
            # "Z"
          }
        }
      }
      event "Path Drawer": Mouse Up {
        n145 = event-data() -> ()  [unwired: 1 in, 4 out]
      }
      event "StartingPosition": Value Change; "StartingPosition": Mouse Down {
        n146 = event-data() -> ()  [unwired: 1 in, 1 out]
        n147 = local read "StartingPosition"() -> (w221:enum16{"1", "2", "3", "4", "No Preset"})
        n148 = Not Equal?(x=enum16{"1", "2", "3", "4", "No Preset"}."No Preset" ("y"), y=w221) -> (x != y?=w226:bool)
        n149 = case shown="True" w226 {
          tunnel: [_ w245] -> w229
          tunnel: w228 -> [_ w244]
          tunnel: w223 -> [_ w242]
          tunnel: w221 -> [_ w231]
          tunnel: w225 -> [_ w236]
          tunnel: w224 -> [_ w235]
          tunnel: w220 -> [_ w234]
          tunnel: dbl[] [1.0, -1.0, 1.0, -1.0] -> [_ w232]
          frame False {
          }
          frame True {
            n150 = Index Array(array=w232, index=w231) -> (element=w230:dbl)
            n151 = Index Array(array=w234, index=w231) -> (element=w233:cluster{u32, u32})
            n152 = Divide(x=w235, y=2.0) -> (x/y=w239:dbl)
            n153 = Multiply(x=w230, y=w239) -> (x*y=w238:dbl)
            n154 = Bundle(w236, w238) -> (w237:cluster{dbl, dbl})  [unwired: 1 in]
            n155 = Add(x=w233, y=w237) -> (x+y=w241:cluster{dbl, dbl})
            n156 = Replace Array Subset(array=w242, new element=w241) -> (w243:cluster{i32, i32}[])  [unwired: 1 in]
            n157 = call "PathToROI.vi"("Path In"=w243, "ROI In"=w244) -> ("ROI Out"=w245:T4)  [unwired: 9 in]
          }
        }
      }
      event "LoadFromLocal": Value Change {
        w271 = T7 {"RobotNeeded"={"Path"=[], "MaxVel"=0.0, "MaxAccel"=0.0, "Backwards?"=FALSE, "PointSpacing"=0.0, "LookaheadDist"=0.0, "Speed/Curve"=1.8, "SlowDistanceAtEnd"=12.0, "SlowSpeed"=15.0}, "Meta"={"Path (px)"=[], "RobotWidth"=0.0, "RobotLength"=0.0, "CenterOfRotYOffset"=0.0, "Roundedness"=0.0, "StartingPositionPreset"=2, "PathName"=""}}  # Data
        n158 = event-data() -> ()  [unwired: 1 in, 2 out]
        n159 = local read "LocalFileNames"() -> (w255:string[])
        n160 = local read "LocalPaths"() -> (w256:i32)
        n161 = Current VI's Path() -> (path=w258:path)
        n162 = Strip Path(path=w258) -> (stripped path=w257:path)  [unwired: 1 out]
        n163 = Build Path(base path=w257, name or relative path="Paths") -> (appended path=w263:path)
        n164 = Index Array(array=w255, index=w256) -> (element=w262:string)
        n165 = Build Path(base path=w263, name or relative path=w262) -> (appended path=w261:path)
        n166 = local write "LoadFromLocal"(FALSE ("Export To File")) -> ()
        n167 = Read from Text File(file (use dialog)=w261) -> (text=w273:string)  [unwired: 3 in, 3 out]
        n168 = Unflatten From JSON(JSON string=w273, type and defaults=w271) -> (value=w270:T7)  [unwired: 5 in, 1 out]
        n169 = Unbundle By Name(w270) -> ("RobotNeeded"=w254:T8, "Meta"=w269:T9)
        n170 = Unbundle By Name(w269) -> ("Path (px)"=w259:cluster{i32, i32}[], "RobotWidth"=w264:dbl, "RobotLength"=w265:dbl, "CenterOfRotYOffset"=w268:dbl, "Roundedness"=w267:dbl, "StartingPositionPreset"=w266:u32)
        n171 = Unbundle By Name(w254) -> ("MaxVel"=w253:dbl, "MaxAccel"=w252:dbl, "Backwards?"=w251:bool, "PointSpacing"=w250:dbl, "LookaheadDist"=w249:dbl, "Speed/Curve"=w248:dbl, "SlowDistanceAtEnd"=w247:dbl, "SlowSpeed"=w246:dbl)
        n172 = call "PathToROI.vi"("Path In"=w259, "ROI In"=w260) -> ("ROI Out"=w274:T4)  [unwired: 9 in]
        n173 = local write "DriveBackwards?"(w251) -> ()
        n174 = local write "MaxVel"(w253) -> ()
        n175 = local write "SlowDistanceAtEnd"(w247) -> ()
        n176 = local write "Roundedness"(w267) -> ()
        n177 = local write "MaxAccel"(w252) -> ()
        n178 = local write "CenterRotOffset"(w268) -> ()
        n179 = local write "Width"(w264) -> ()
        n180 = local write "Length"(w265) -> ()
        n181 = local write "SlowSpeed"(w246) -> ()
        n182 = local write "StartingPosition"(w266) -> ()
        n183 = local write "Lookahead"(w249) -> ()
        n184 = local write "Speed/Curve"(w248) -> ()
        n185 = local write "PointSpacing"(w250) -> ()
      }
      event "Flip Path": Value Change {
        w283 = cluster{i32, i32} {0, 203}
        # "Center of field"
        n186 = event-data() -> ()  [unwired: 1 in, 2 out]
        n187 = local read "StartingPosition"() -> (w277:enum16{"1", "2", "3", "4", "No Preset"})
        n188 = local write "Flip Path"(FALSE ("Export To File")) -> ()
        n189 = Not Equal?(x=enum16{"1", "2", "3", "4", "No Preset"}."No Preset", y=w277) -> (x != y?=w278:bool)
        n190 = Subtract(x=w281, y=w283) -> (x-y=w282:cluster{i32, i32}[])
        n191 = case shown="True" w278 {
          tunnel: w277 -> [w289 w292]
          tunnel: [w289 w290] -> w276
          frame False {
          }
          frame True {
            n192 = Subtract(x=3, y=w292) -> (x-y=w290:i32)
          }
        }
        n193 = Multiply(x=w282, y=cluster{i32, i32} {1, -1}) -> (x*y=w284:cluster{i32, i32}[])
        n194 = Add(x=w284, y=w283) -> (x+y=w280:cluster{i32, i32}[])
        n195 = call "PathToROI.vi"("Path In"=w280, "ROI In"=w287) -> ("ROI Out"=w286:T4)  [unwired: 9 in]
        n196 = local write "StartingPosition"(w276) -> ()
      }
    }
    n197 = Unbundle By Name(w33) -> ("Global Rectangle"=w57:i32[])
    n198 = Empty Array?(array=w57) -> (empty?=w56:bool)
    n199 = case shown="False" w56 {
      tunnel: w33 -> [w74 _]
      frame False {
        n200 = property on="Path Drawer" class="ImageControl"("ROI"=w74) -> (error out=w75:errorcluster)  [unwired: 2 in, 1 out]
        n201 = call <vilib>:"Clear Errors.vi"("error in (no error)"=w75) -> ()  [unwired: 5 in, 2 out]
      }
      frame True {
      }
    }
  }
